vi "for.vi"() -> ()   [LabVIEW 2020]
panel:
  out "number (0 to 1)":dbl
  in  "Numero de I":i32
  out "I":i32
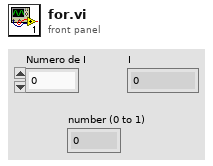
[diagram p1: front panel]
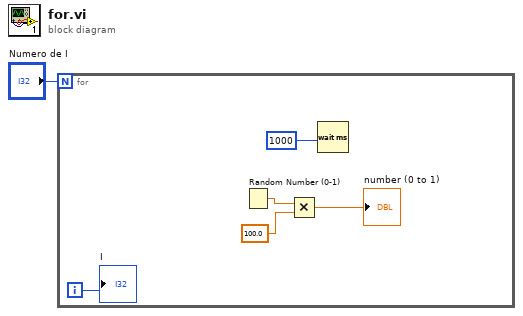
[diagram p0: block diagram]
diagram:
  n1 = for {
    N: "Numero de I" -> [_]
    i -> [w6]
    n2 = Random Number (0-1)() -> (number: 0 to 1=w5:dbl)
    n3 = Multiply(x=w5, y=100.0) -> (x*y=→"number (0 to 1)":dbl)
    n4 = Wait (ms)(milliseconds to wait=1000) -> ()  [unwired: 1 out]
    "I" <- w6
  }
